vi "SetLabel.vi"(8 "error in (no error)":errorcluster caption="错误输入（无错误）", 11 "TPlot 输入":refnum<class "TPlot.lvclass">) -> (0 "error out":errorcluster caption="错误输出", 3 "TPlot 输出":refnum<class "TPlot.lvclass">)   [LabVIEW 2018, in "DataDisplay.lvlib" / "TPlot.lvclass"]
uses:
  TPlot.lvclass
  TPlot.lvclass/TPlot.ctl
  SubVI/DD_Parameter.vi
  DataDisplay.lvlib
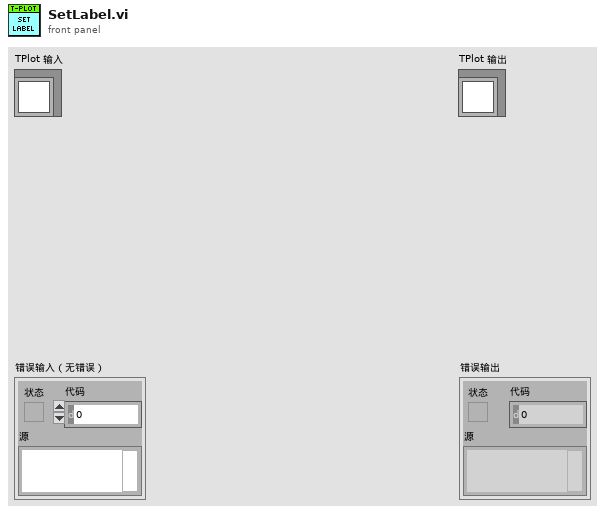
[diagram p1: front panel]
types:
  T1 = typedef "DataDisplay.lvlib/DD_ChannelInfo.ctl" = cluster{"名称":string, "单位":string, "数据类型":enum16{"Real", "Int"}, "趋势线":enum16{"N/A", "X", "Y"}}
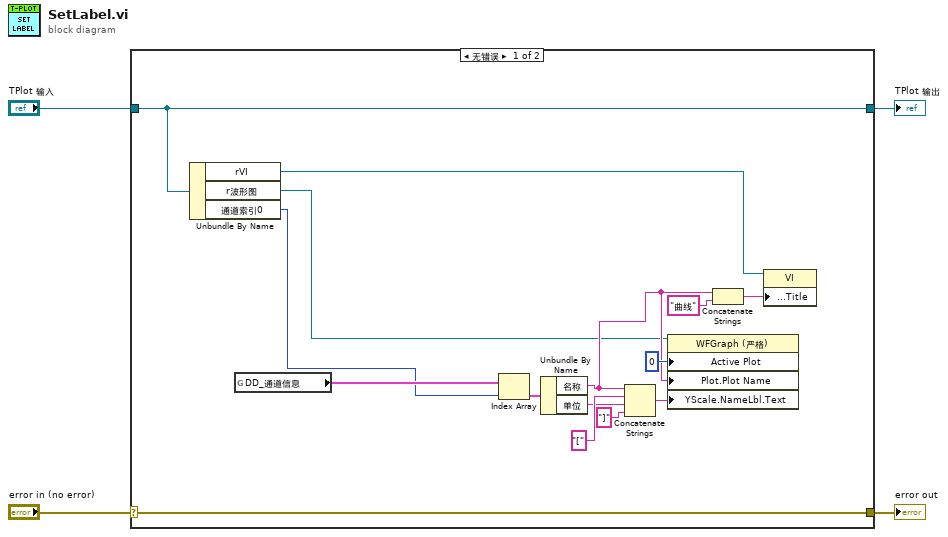
[diagram p0: block diagram]
diagram:
  n1 = case shown="无错误" "error in (no error)" {
    selector: "error in (no error)" -> [w19 w21]
    tunnel: [w19 w21] -> w3
    tunnel: [w9 w20] -> w1
    tunnel: "TPlot 输入" -> [w9 w20]
    frame No Error {
      n2 = Unbundle By Name(w9) -> ("rVI"=w7:refnum<vi>, "r波形图"=w6:refnum<vi>, "通道索引0"=w5:i32)
      n3 = global read "DD_Parameter.vi" "DD_通道信息"() -> (w10:T1[])
      n4 = Index Array(array=w10, index=w5) -> (element=w16:T1)
      n5 = Unbundle By Name(w16) -> ("名称"=w8:string, "单位"=w14:string)
      n6 = Concatenate Strings(w8, "[" ("字符串"), w14, "]" ("字符串")) -> (w12:string)
      n7 = property class="WFGraph (严格)"(reference=w6, "Active Plot"=u32 0 ("活动曲线"), "Plot.Plot Name"=w8, "YScale.NameLbl.Text"=w12) -> ()  [unwired: 1 in, 2 out]
      n8 = Concatenate Strings(w8, "曲线" ("字符串")) -> (w17:string)
      n9 = property class="VI"(reference=w7, "Front Panel.Title"=w17) -> ()  [unwired: 1 in, 2 out]
    }
    frame Error {
    }
  }
  "error out" <- w3
  "TPlot 输出" <- w1
